vi "Autonomous Independent.vi"() -> ()   [LabVIEW 2016]
doc: "This VI is called when autonomous begins, and will automatically be terminated when autonomous ends. You can carry out timed or sensor driven robot movement independently without needing to return to the caller."
uses:
  <vilib>/Rock Robotics/Network Tables/NT Read Number.vi
  Robot Global Data.vi
  <vilib>/addons/control/pid/pid.llb/PID (DBL).vi
  <vilib>/Rock Robotics/Network Tables/NT Write Number.vi
  <vilib>/addons/control/pid/NI_PID_pid.lvlib
panel:
  out "Distance 9-2":dbl
  out "Distance 9 - 1":dbl
  out "Distance 1":dbl
  out "Distance 2":dbl
  out "Gyro Angle 4":dbl(knob) scale=0.0..360.0
  out "Gyro Zero angle":dbl
  out "Boolean 2":bool
  out "Current 2":dbl=14.75
  out "Elapsed Time (s) 2":dbl caption="Elapsed Time (s)"
  out "Boolean 9":bool
  out "Gyro Angle 4":dbl(knob) scale=0.0..360.0
  out "Numeric 2":dbl
  out "drive current 2":dbl=2.75
  out "Gyro Angle 3":dbl(knob) scale=0.0..360.0
  out "Distance 2":dbl
  out "Distance":dbl
  out "Boolean":bool
  out "Current":dbl=14.75
  out "Elapsed Time (s)":dbl
  out "Boolean 8":bool
  out "Gyro Angle 3":dbl(knob) scale=0.0..360.0
  out "Numeric":dbl
  out "drive current":dbl=2.75
  out "Gyro Angle 2":dbl(knob) scale=0.0..360.0
  out "abs(x)":dbl
  out "Loop Speed":u32
  in  "Manual Auto Select":bool
  in  "Auto Select":T1(ring)=enum."baseline"
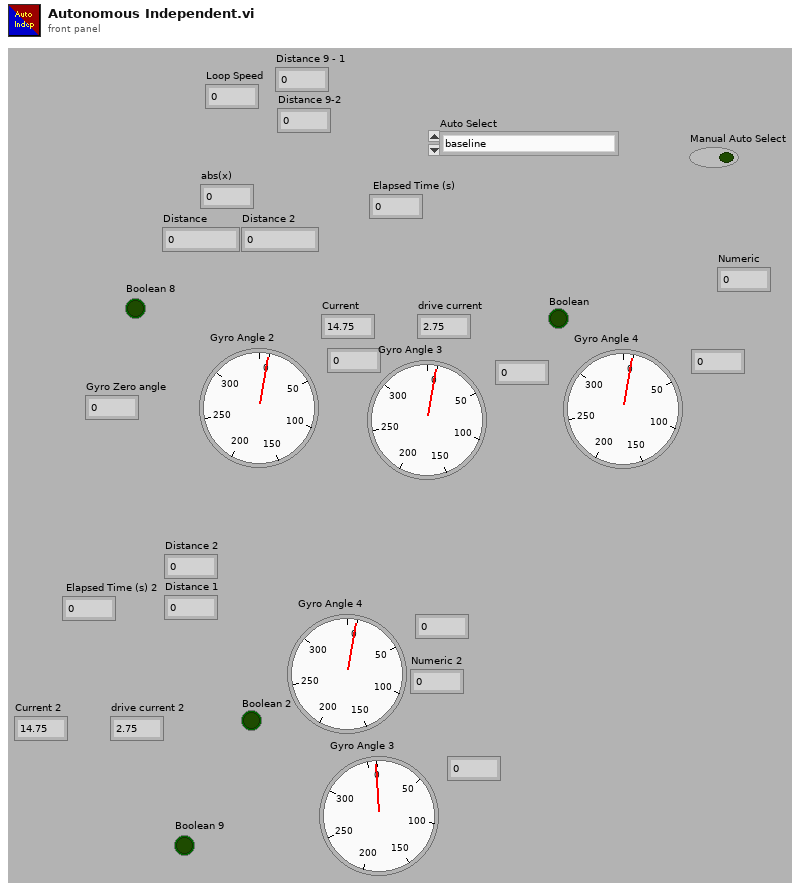
[diagram p1: front panel]
types:
  T1 = enum16{"default", "baseline", "center gear", "left gear", "right gear", "10 shoot then gear prep blue", "10 shoot then gear prep red", "Blank", "move to shoot red", "hopper shoot bue", "hopper shoot red"}
  T2 = cluster{"proportional gain (Kc)":dbl, "integral time (Ti, min)":dbl, "derivative time (Td, min)":dbl}
  T3 = typedef "WPI_EncoderDevRef.ctl" = cluster{"DevStatus":errorcluster, "EncoderIndex":T4, "CounterIndex":T5, "DistancePerCount":dbl, "Decoding Type":T6}
  T4 = typedef "FPGA_EncoderIdx.ctl" = enum8{"Enc 0", "Enc 1", "Enc 2", "Enc 3", "Enc 4", "Enc 5", "Enc 6", "Enc 7", "Invalid"}
  T5 = typedef "FPGA_CounterCtrSystemIndex.ctl" = enum8{"Ctr 0", "Ctr 1", "Ctr 2", "Ctr 3", "Ctr 4", "Ctr 5", "Ctr 6", "Ctr 7", "Invalid"}
  T6 = typedef "WPI_EncoderType.ctl" = enum16{"1x", "2x", "4x"}
  T7 = typedef "WPI_MotorControlDeviceRef.ctl" = cluster{"DeviceStatus":errorcluster, "Type":T8, "PWM":cluster{"PWM Channel":T9, "DeadBand":T10}, "CAN":cluster{"Device Number":u8, "SetOutput VI Ref":variant, "GetOutput VI Ref":variant, "Enable VI Ref":variant, "Disable VI Ref":variant, "Data":variant}, "Invert":bool}
  T8 = typedef "WPI_MotorControlType.ctl" = enum16{"PWM", "CAN"}
  T9 = typedef "FPGA_DIOPWMChannel.ctl" = enum8{"PWM 0", "PWM 1", "PWM 2", "PWM 3", "PWM 4", "PWM 5", "PWM 6", "PWM 7", "PWM 8", "PWM 9", "PWM MXP 0", "PWM MXP 1", "PWM MXP 2", "PWM MXP 3", "PWM MXP 4", "PWM MXP 5", "PWM MXP 6", "PWM MXP 7", "PWM MXP 8", "PWM MXP 9", "Invalid"}
  T10 = typedef "WPI_PWMDeadband.ctl" = cluster{"Name":string, "maxPositivePwm":i32, "minPositivePwm":i32, "centerPwm":i32, "maxNegativePwm":i32, "minNegativePwm":i32, "angularRange":u16}
  T11 = typedef "WPI_CANTalonSRX_GlobalStatus.ctl" = cluster{"Applied Throttle":dbl, "Module Enabled":bool, "CAN Error":errorcluster, "Closed Loop Error":dbl, "Forward Limit Switch Closed":bool, "Reverse Limit Switch Closed":bool, "Sensor Position":dbl, "Sensor Velocity":dbl, "Current":dbl, "Sticky Fault - Over Temp":bool, "Sticky Fault - Under Voltage":bool, "Sticky Fault - Forward Limit":bool, "Sticky Fault - Reverse Limit":bool, "Sticky Fault - Forward Soft Limit":bool, "Sticky Fault - Reverse Soft Limit":bool, "Brake is Enabled":bool, "Encoder Position":dbl, "Encoder Velocity":dbl, "Encoder Index Count":dbl, "Encoder A Pin State":bool, "Encoder B Pin State":bool, "Encoder Index Pin State":bool, "Analog In":dbl, "Analog In Velocity":dbl, "Temperature (C)":dbl, "Battery Voltage":dbl, "Control 5 Is Supported":bool, "Current Profile Slot Select":dbl, "Pos Div 8":bool, "Vel Div 4":bool, "Pulse Width Position":i32, "Pulse Width Velocity":i32, "Pulse Width Rise To Rise (us)":i32, "Pulse Width Rise To Fall (us)":i32, "Mot Prof Active Is Under Run":bool, "Mot Prof Active Has Under Run":bool, "Mot Prof Active Is Last":bool, "Mot Prof Active Velocity Only":bool, "Mot Prof Active Is Valid":bool, "Mot Prof Buffer Is Full":bool, "Mot Prof Active Profile Slot Select":i32, "Mot Prof NextID":i32, "Mot Prof Count":i32, "Mot Prof Active Velocity":dbl, "Mot Prof Active Position":dbl, "Mot Prof Output Enable":i32, "UsageFrame":u32, "Motion Magic Active Trajectory":cluster{"Velocity":dbl, "Position":dbl}}
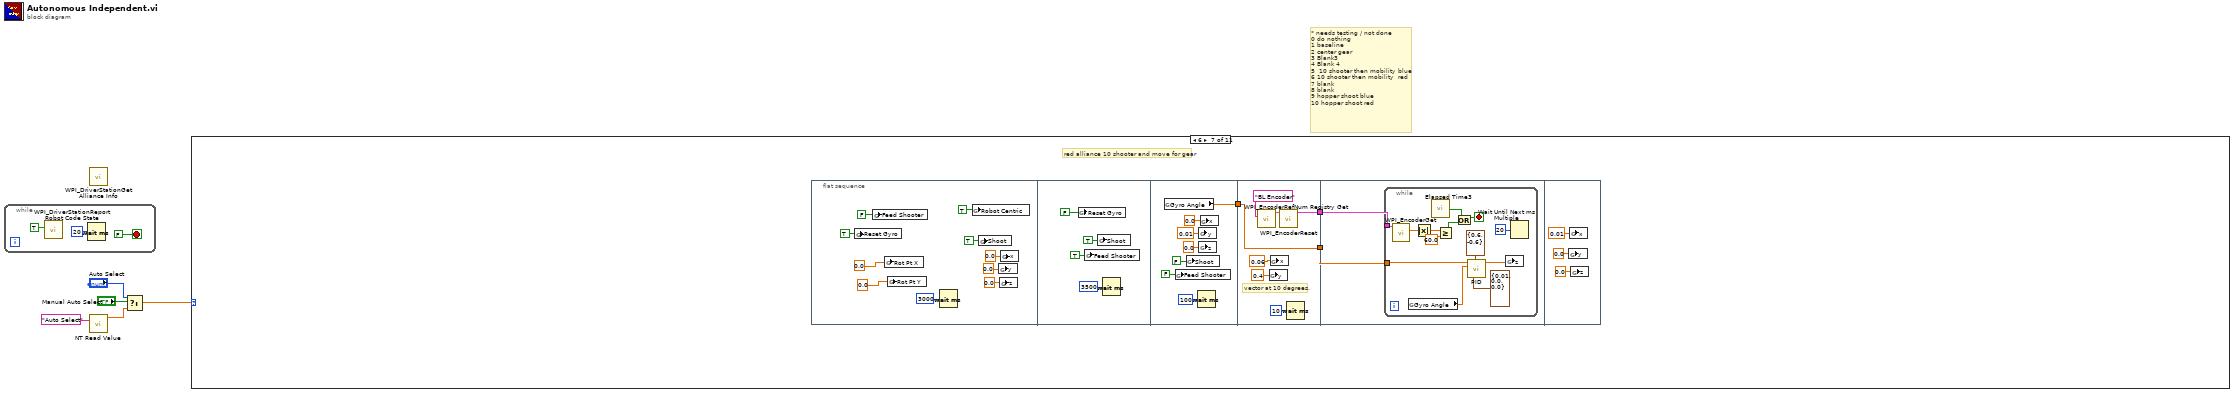
[diagram p0: block diagram]
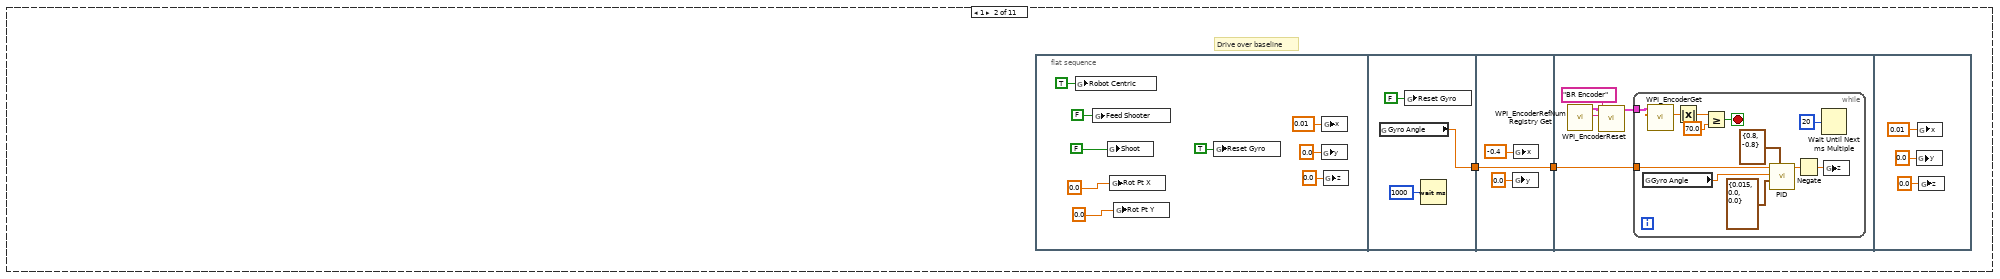
[diagram p3: hidden frame]
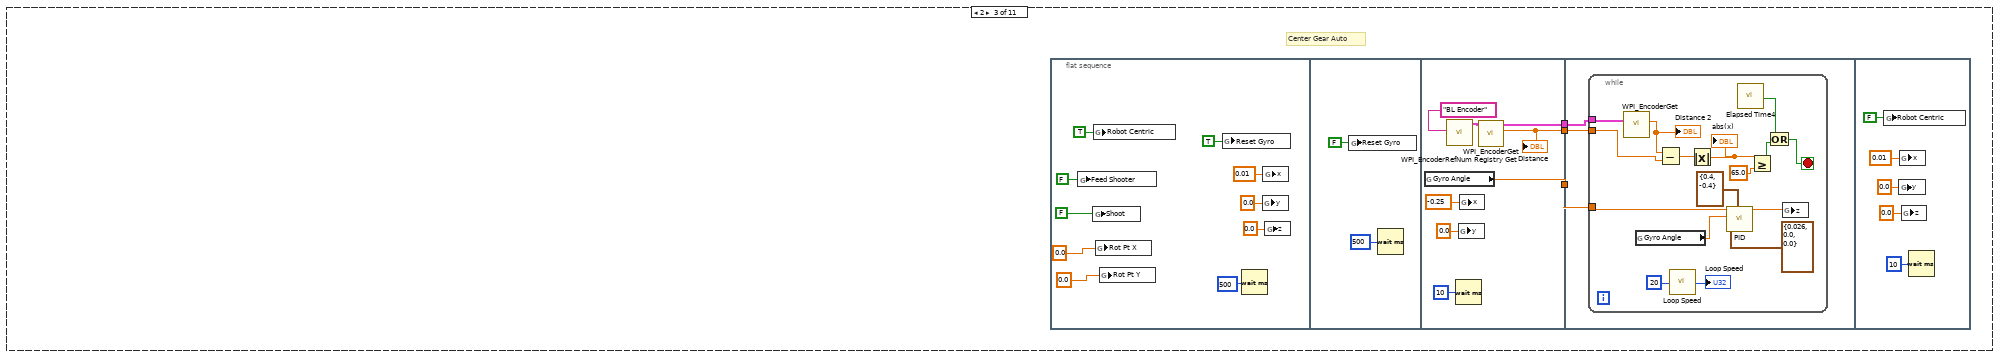
[diagram p4: hidden frame]
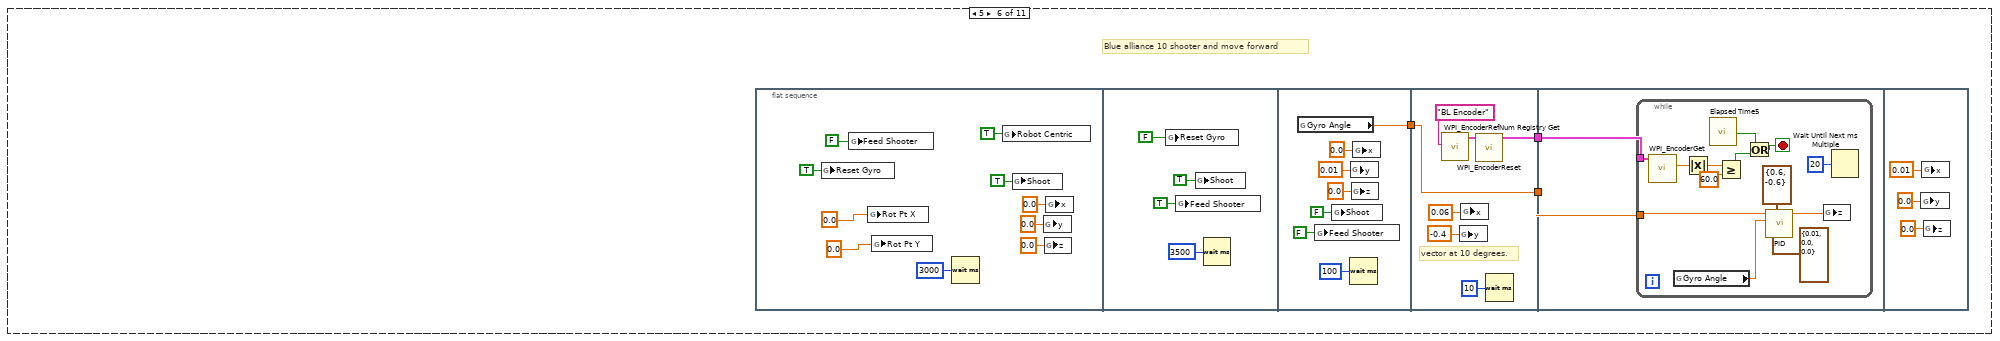
[diagram p7: hidden frame]
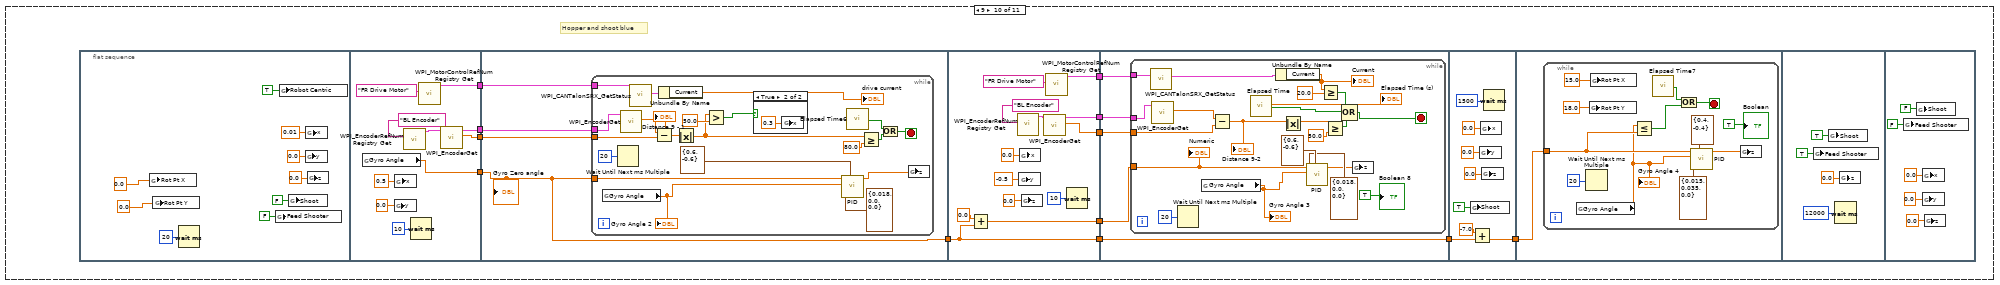
[diagram p10: hidden frame]
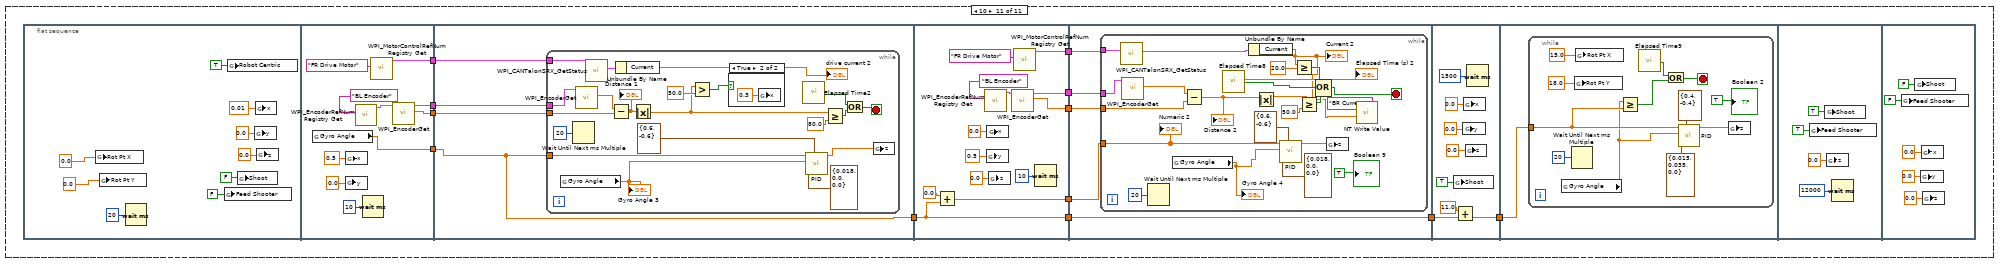
[diagram p12: hidden frame]
diagram:
  # "* needs testing / not done\n0 do nothing\n1 baseline\n2 center gear\n3 Blank3\n4 Blank 4\n5  10 shooter then mobility blue \n6 10 shooter then mobility  red\n7 blank\n8 blank\n9 hopper shoot blue\n10 hopper shoot red"
  n1 = while {
    stop <- FALSE stop-if-true
    n2 = call <vilib>:"WPI_DriverStationReport Robot Code State.vi"("Autonomous"=TRUE) -> ()  [unwired: 10 in, 1 out]
    n3 = Wait (ms)(milliseconds to wait=u32 20) -> ()  [unwired: 1 out]
  }
  n4 = call-poly <vilib>:"NT Read Value.vi"("Name"="Auto Select") -> ("Numeric"=w1:dbl)  [unwired: 9 in, 1 out]
  n5 = call <vilib>:"WPI_DriverStationGet Alliance Info.vi"() -> ()  [unwired: 12 out]
  n6 = Select(t="Auto Select", s="Manual Auto Select", f=w1) -> (s? t:f=w5:dbl)
  n7 = case shown="6" w5 {
    frame 0, Default {
    }
    frame 1 {
      # "Drive over baseline"
      n8 = flat-sequence {
        tunnel: [w21] -> w9
        tunnel: [w23] -> w10
        tunnel: w9 -> [w23]
        tunnel: w10 -> [w26]
        frame #0 {
          n9 = global write "Robot Global Data.vi" "Robot Centric"(TRUE ("Robot Centric")) -> ()
          n10 = global write "Robot Global Data.vi" "Feed Shooter"(FALSE ("Robot Centric")) -> ()
          n11 = global write "Robot Global Data.vi" "Shoot"(FALSE ("Robot Centric")) -> ()
          n12 = global write "Robot Global Data.vi" "Rot Pt X"(0.0 ("Rot Pt X")) -> ()
          n13 = global write "Robot Global Data.vi" "Rot Pt Y"(0.0 ("Rot Pt X")) -> ()
          n14 = global write "Robot Global Data.vi" "Reset Gyro"(TRUE ("Reset Gyro")) -> ()
          n15 = global write "Robot Global Data.vi" "y"(0.0 ("y")) -> ()
          n16 = global write "Robot Global Data.vi" "x"(0.01 ("x")) -> ()
          n17 = global write "Robot Global Data.vi" "z"(0.0 ("z")) -> ()
        }
        frame #1 {
          n18 = global read "Robot Global Data.vi" "Gyro Angle"() -> (w21:dbl)
          n19 = global write "Robot Global Data.vi" "Reset Gyro"(FALSE ("Reset Gyro")) -> ()
          n20 = Wait (ms)(milliseconds to wait=u32 1000) -> ()  [unwired: 1 out]
        }
        frame #2 {
          n21 = global write "Robot Global Data.vi" "y"(0.0 ("y")) -> ()
          n22 = global write "Robot Global Data.vi" "x"(-0.4 ("x")) -> ()
        }
        frame #3 {
          n23 = call <vilib>:"WPI_EncoderRefNum Registry Get.vi"("refnum name"="BR Encoder") -> ("EncoderDevRef"=w28:T3)  [unwired: 9 in, 1 out]
          n24 = call <vilib>:"WPI_EncoderReset.vi"("EncoderDevRef"=w28) -> ("EncoderDevRef"=w27:T3)  [unwired: 9 in, 1 out]
          n25 = while {
            tunnel: w27 -> [w41]
            tunnel: w26 -> [w32]
            stop <- w39 stop-if-true
            n26 = global read "Robot Global Data.vi" "Gyro Angle"() -> (w31:dbl)
            n27 = call <vilib>:"WPI_EncoderGet.vi"("EncoderDevRef"=w41) -> ("Distance"=w40:dbl)  [unwired: 5 in, 5 out]
            n28 = Absolute Value(x=w40) -> (abs(x)=w34:dbl)
            n29 = Greater Or Equal?(x=w34, y=70.0) -> (x >= y?=w39:bool)
            n30 = call-poly <vilib>:"PID.vi"("output range"=cluster{"output high":dbl, "output low":dbl} {"output high"=0.8, "output low"=-0.8}, "PID gains"=T2 {"proportional gain (Kc)"=0.015, "integral time (Ti, min)"=0.0, "derivative time (Td, min)"=0.0} ("PID gains 2"), "process variable"=w31, "setpoint"=w32) -> ("output"=w37:dbl)  [unwired: 6 in, 1 out]
            n31 = Negate(x=w37) -> (-x=w35:dbl)
            n32 = Wait Until Next ms Multiple(millisecond multiple=u32 20) -> ()  [unwired: 1 out]
            n33 = global write "Robot Global Data.vi" "z"(w35) -> ()
          }
        }
        frame #4 {
          n34 = global write "Robot Global Data.vi" "y"(0.0 ("y")) -> ()
          n35 = global write "Robot Global Data.vi" "x"(0.01 ("x")) -> ()
          n36 = global write "Robot Global Data.vi" "z"(0.0 ("z")) -> ()
        }
      }
    }
    frame 2 {
      # "Center Gear Auto"
      n37 = flat-sequence {
        tunnel: [w65] -> w47
        tunnel: [w61] -> w46
        tunnel: [w60] -> w45
        tunnel: w47 -> [w70]
        tunnel: w46 -> [w69]
        tunnel: w45 -> [w68]
        frame #0 {
          n38 = global write "Robot Global Data.vi" "Feed Shooter"(FALSE ("Robot Centric")) -> ()
          n39 = global write "Robot Global Data.vi" "Shoot"(FALSE ("Robot Centric")) -> ()
          n40 = global write "Robot Global Data.vi" "Robot Centric"(TRUE ("Robot Centric")) -> ()
          n41 = global write "Robot Global Data.vi" "Rot Pt X"(0.0 ("Rot Pt X")) -> ()
          n42 = global write "Robot Global Data.vi" "Rot Pt Y"(0.0 ("Rot Pt X")) -> ()
          n43 = global write "Robot Global Data.vi" "Reset Gyro"(TRUE ("Reset Gyro")) -> ()
          n44 = Wait (ms)(milliseconds to wait=u32 500) -> ()  [unwired: 1 out]
          n45 = global write "Robot Global Data.vi" "y"(0.0 ("y")) -> ()
          n46 = global write "Robot Global Data.vi" "x"(0.01 ("x")) -> ()
          n47 = global write "Robot Global Data.vi" "z"(0.0 ("z")) -> ()
        }
        frame #1 {
          n48 = global write "Robot Global Data.vi" "Reset Gyro"(FALSE ("Reset Gyro")) -> ()
          n49 = Wait (ms)(milliseconds to wait=u32 500) -> ()  [unwired: 1 out]
        }
        frame #2 {
          n50 = global read "Robot Global Data.vi" "Gyro Angle"() -> (w65:dbl)
          n51 = call <vilib>:"WPI_EncoderRefNum Registry Get.vi"("refnum name"="BL Encoder") -> ("EncoderDevRef"=w63:T3)  [unwired: 9 in, 1 out]
          n52 = Wait (ms)(milliseconds to wait=u32 10) -> ()  [unwired: 1 out]
          n53 = global write "Robot Global Data.vi" "y"(0.0 ("y")) -> ()
          n54 = global write "Robot Global Data.vi" "x"(-0.25 ("x")) -> ()
          n55 = call <vilib>:"WPI_EncoderGet.vi"("EncoderDevRef"=w63) -> ("Distance"=w60:dbl, "EncoderDevRef"=w61:T3)  [unwired: 5 in, 4 out]
          "Distance" <- w60
        }
        frame #3 {
          n56 = while {
            tunnel: w69 -> [w86]
            tunnel: w70 -> [w83]
            tunnel: w68 -> [w76]
            stop <- w71 stop-if-true
            n57 = call <vilib>:"WPI_EncoderGet.vi"("EncoderDevRef"=w86) -> ("Distance"=w77:dbl)  [unwired: 5 in, 5 out]
            "Distance 2" <- w77
            n58 = global read "Robot Global Data.vi" "Gyro Angle"() -> (w81:dbl)
            n59 = Subtract(x=w77, y=w76) -> (x-y=w75:dbl)
            n60 = call "Loop Speed.vi"("milliseconds to wait"=u32 20) -> ("Loop Speed"=→"Loop Speed":u32)
            n61 = Absolute Value(x=w75) -> (abs(x)=w74:dbl)
            "abs(x)" <- w74
            n62 = call-poly <vilib>:"PID.vi"("output range"=cluster{"output high":dbl, "output low":dbl} {"output high"=0.4, "output low"=-0.4}, "PID gains"=T2 {"proportional gain (Kc)"=0.026, "integral time (Ti, min)"=0.0, "derivative time (Td, min)"=0.0}, "process variable"=w81, "setpoint"=w83) -> ("output"=w79:dbl)  [unwired: 6 in, 1 out]
            n63 = call "Elapsed Time4"() -> ("Time has Elapsed"=w72:bool)  [unwired: 12 in, 7 out]
            n64 = Greater Or Equal?(x=w74, y=65.0) -> (x >= y?=w73:bool)
            n65 = Or(x=w72, y=w73) -> (x .or. y?=w71:bool)
            n66 = global write "Robot Global Data.vi" "z"(w79) -> ()
          }
        }
        frame #4 {
          n67 = global write "Robot Global Data.vi" "Robot Centric"(FALSE ("Robot Centric")) -> ()
          n68 = global write "Robot Global Data.vi" "y"(0.0 ("y")) -> ()
          n69 = global write "Robot Global Data.vi" "x"(0.01 ("x")) -> ()
          n70 = global write "Robot Global Data.vi" "z"(0.0 ("z")) -> ()
          n71 = Wait (ms)(milliseconds to wait=u32 10) -> ()  [unwired: 1 out]
        }
      }
    }
    frame 3 {
      # "find current of drive motors when\n they have more than normal load\n and use that as a safe stop"
    }
    frame 4 {
    }
    frame 5 {
      # "Blue alliance 10 shooter and move forward"
      n72 = flat-sequence {
        tunnel: [w109] -> w93
        tunnel: [w120] -> w94
        tunnel: w93 -> [w120]
        tunnel: [w117] -> w92
        tunnel: w94 -> [w124]
        tunnel: w92 -> [w123]
        frame #0 {
          n73 = global write "Robot Global Data.vi" "Reset Gyro"(TRUE ("Reset Gyro")) -> ()
          n74 = global write "Robot Global Data.vi" "Feed Shooter"(FALSE ("Robot Centric")) -> ()
          n75 = global write "Robot Global Data.vi" "Rot Pt X"(0.0 ("Rot Pt X")) -> ()
          n76 = global write "Robot Global Data.vi" "Rot Pt Y"(0.0 ("Rot Pt X")) -> ()
          n77 = Wait (ms)(milliseconds to wait=u32 3000) -> ()  [unwired: 1 out]
          n78 = global write "Robot Global Data.vi" "Robot Centric"(TRUE ("Robot Centric")) -> ()
          n79 = global write "Robot Global Data.vi" "Shoot"(TRUE ("Shoot")) -> ()
          n80 = global write "Robot Global Data.vi" "y"(0.0 ("y")) -> ()
          n81 = global write "Robot Global Data.vi" "z"(0.0 ("z")) -> ()
          n82 = global write "Robot Global Data.vi" "x"(0.0 ("x")) -> ()
        }
        frame #1 {
          n83 = global write "Robot Global Data.vi" "Reset Gyro"(FALSE ("Reset Gyro")) -> ()
          n84 = global write "Robot Global Data.vi" "Feed Shooter"(TRUE ("Feed Shooter")) -> ()
          n85 = global write "Robot Global Data.vi" "Shoot"(TRUE ("Shoot")) -> ()
          n86 = Wait (ms)(milliseconds to wait=u32 3500) -> ()  [unwired: 1 out]
        }
        frame #2 {
          n87 = global read "Robot Global Data.vi" "Gyro Angle"() -> (w109:dbl)
          n88 = global write "Robot Global Data.vi" "Feed Shooter"(FALSE ("Feed Shooter")) -> ()
          n89 = global write "Robot Global Data.vi" "Shoot"(FALSE ("Shoot")) -> ()
          n90 = Wait (ms)(milliseconds to wait=u32 100) -> ()  [unwired: 1 out]
          n91 = global write "Robot Global Data.vi" "y"(0.01 ("y")) -> ()
          n92 = global write "Robot Global Data.vi" "z"(0.0 ("z")) -> ()
          n93 = global write "Robot Global Data.vi" "x"(0.0 ("x")) -> ()
        }
        frame #3 {
          # "vector at 10 degrees."
          n94 = call <vilib>:"WPI_EncoderRefNum Registry Get.vi"("refnum name"="BL Encoder") -> ("EncoderDevRef"=w118:T3)  [unwired: 9 in, 1 out]
          n95 = global write "Robot Global Data.vi" "y"(-0.4 ("y")) -> ()
          n96 = global write "Robot Global Data.vi" "x"(0.06 ("x")) -> ()
          n97 = call <vilib>:"WPI_EncoderReset.vi"("EncoderDevRef"=w118) -> ("EncoderDevRef"=w117:T3)  [unwired: 9 in, 1 out]
          n98 = Wait (ms)(milliseconds to wait=u32 10) -> ()  [unwired: 1 out]
        }
        frame #4 {
          n99 = while {
            tunnel: w123 -> [w137]
            tunnel: w124 -> [w133]
            stop <- w128 stop-if-true
            n100 = call <vilib>:"WPI_EncoderGet.vi"("EncoderDevRef"=w137) -> ("Distance"=w136:dbl)  [unwired: 5 in, 5 out]
            n101 = global read "Robot Global Data.vi" "Gyro Angle"() -> (w130:dbl)
            n102 = Absolute Value(x=w136) -> (abs(x)=w132:dbl)
            n103 = call "Elapsed Time5"() -> ("Time has Elapsed"=w126:bool)  [unwired: 12 in, 7 out]
            n104 = Greater Or Equal?(x=w132, y=60.0 ("Distance to travel")) -> (x >= y?=w127:bool)
            n105 = Or(x=w126, y=w127) -> (x .or. y?=w128:bool)
            n106 = call-poly <vilib>:"PID.vi"("output range"=cluster{"output high":dbl, "output low":dbl} {"output high"=0.6, "output low"=-0.6}, "PID gains"=T2 {"proportional gain (Kc)"=0.01, "integral time (Ti, min)"=0.0, "derivative time (Td, min)"=0.0}, "process variable"=w130, "setpoint"=w133) -> ("output"=w125:dbl)  [unwired: 6 in, 1 out]
            n107 = global write "Robot Global Data.vi" "z"(w125) -> ()
            n108 = Wait Until Next ms Multiple(millisecond multiple=u32 20) -> ()  [unwired: 1 out]
          }
        }
        frame #5 {
          n109 = global write "Robot Global Data.vi" "y"(0.0 ("y")) -> ()
          n110 = global write "Robot Global Data.vi" "x"(0.01 ("x")) -> ()
          n111 = global write "Robot Global Data.vi" "z"(0.0 ("z")) -> ()
        }
      }
    }
    frame 6 {
      # "red alliance 10 shooter and move for gear"
      n112 = flat-sequence {
        tunnel: [w158] -> w143
        tunnel: [w169] -> w142
        tunnel: w143 -> [w169]
        tunnel: [w166] -> w141
        tunnel: w142 -> [w172]
        tunnel: w141 -> [w173]
        frame #0 {
          n113 = global write "Robot Global Data.vi" "Reset Gyro"(TRUE ("Reset Gyro")) -> ()
          n114 = global write "Robot Global Data.vi" "Feed Shooter"(FALSE ("Robot Centric")) -> ()
          n115 = global write "Robot Global Data.vi" "Rot Pt X"(0.0 ("Rot Pt X")) -> ()
          n116 = global write "Robot Global Data.vi" "Rot Pt Y"(0.0 ("Rot Pt X")) -> ()
          n117 = Wait (ms)(milliseconds to wait=u32 3000) -> ()  [unwired: 1 out]
          n118 = global write "Robot Global Data.vi" "Robot Centric"(TRUE ("Robot Centric")) -> ()
          n119 = global write "Robot Global Data.vi" "Shoot"(TRUE ("Shoot")) -> ()
          n120 = global write "Robot Global Data.vi" "y"(0.0 ("y")) -> ()
          n121 = global write "Robot Global Data.vi" "z"(0.0 ("z")) -> ()
          n122 = global write "Robot Global Data.vi" "x"(0.0 ("x")) -> ()
        }
        frame #1 {
          n123 = global write "Robot Global Data.vi" "Reset Gyro"(FALSE ("Reset Gyro")) -> ()
          n124 = global write "Robot Global Data.vi" "Feed Shooter"(TRUE ("Feed Shooter")) -> ()
          n125 = global write "Robot Global Data.vi" "Shoot"(TRUE ("Shoot")) -> ()
          n126 = Wait (ms)(milliseconds to wait=u32 3500) -> ()  [unwired: 1 out]
        }
        frame #2 {
          n127 = global read "Robot Global Data.vi" "Gyro Angle"() -> (w158:dbl)
          n128 = global write "Robot Global Data.vi" "Feed Shooter"(FALSE ("Feed Shooter")) -> ()
          n129 = global write "Robot Global Data.vi" "Shoot"(FALSE ("Shoot")) -> ()
          n130 = Wait (ms)(milliseconds to wait=u32 100) -> ()  [unwired: 1 out]
          n131 = global write "Robot Global Data.vi" "y"(0.01 ("y")) -> ()
          n132 = global write "Robot Global Data.vi" "z"(0.0 ("z")) -> ()
          n133 = global write "Robot Global Data.vi" "x"(0.0 ("x")) -> ()
        }
        frame #3 {
          # "vector at 10 degrees."
          n134 = call <vilib>:"WPI_EncoderRefNum Registry Get.vi"("refnum name"="BL Encoder") -> ("EncoderDevRef"=w167:T3)  [unwired: 9 in, 1 out]
          n135 = global write "Robot Global Data.vi" "y"(0.4 ("y")) -> ()
          n136 = global write "Robot Global Data.vi" "x"(0.06 ("x")) -> ()
          n137 = call <vilib>:"WPI_EncoderReset.vi"("EncoderDevRef"=w167) -> ("EncoderDevRef"=w166:T3)  [unwired: 9 in, 1 out]
          n138 = Wait (ms)(milliseconds to wait=u32 10) -> ()  [unwired: 1 out]
        }
        frame #4 {
          n139 = while {
            tunnel: w173 -> [w186]
            tunnel: w172 -> [w182]
            stop <- w177 stop-if-true
            n140 = call <vilib>:"WPI_EncoderGet.vi"("EncoderDevRef"=w186) -> ("Distance"=w185:dbl)  [unwired: 5 in, 5 out]
            n141 = global read "Robot Global Data.vi" "Gyro Angle"() -> (w179:dbl)
            n142 = Absolute Value(x=w185) -> (abs(x)=w181:dbl)
            n143 = call "Elapsed Time3"() -> ("Time has Elapsed"=w175:bool)  [unwired: 12 in, 7 out]
            n144 = Greater Or Equal?(x=w181, y=60.0 ("Distance to travel")) -> (x >= y?=w176:bool)
            n145 = Or(x=w175, y=w176) -> (x .or. y?=w177:bool)
            n146 = call-poly <vilib>:"PID.vi"("output range"=cluster{"output high":dbl, "output low":dbl} {"output high"=0.6, "output low"=-0.6}, "PID gains"=T2 {"proportional gain (Kc)"=0.01, "integral time (Ti, min)"=0.0, "derivative time (Td, min)"=0.0}, "process variable"=w179, "setpoint"=w182) -> ("output"=w174:dbl)  [unwired: 6 in, 1 out]
            n147 = global write "Robot Global Data.vi" "z"(w174) -> ()
            n148 = Wait Until Next ms Multiple(millisecond multiple=u32 20) -> ()  [unwired: 1 out]
          }
        }
        frame #5 {
          n149 = global write "Robot Global Data.vi" "y"(0.0 ("y")) -> ()
          n150 = global write "Robot Global Data.vi" "x"(0.01 ("x")) -> ()
          n151 = global write "Robot Global Data.vi" "z"(0.0 ("z")) -> ()
        }
      }
    }
    frame 7 {
    }
    frame 8 {
    }
    frame 9 {
      # "Hopper and shoot blue"
      n152 = flat-sequence {
        tunnel: [w219] -> w194
        tunnel: [w213] -> w193
        tunnel: [w212] -> w192
        tunnel: [w211] -> w191
        tunnel: w194 -> [w224]
        tunnel: [w224] -> w201
        tunnel: w193 -> [w223]
        tunnel: w192 -> [w222]
        tunnel: w191 -> [w221]
        tunnel: w201 -> [w256]
        tunnel: [w257] -> w200
        tunnel: [w256] -> w199
        tunnel: [w249] -> w196
        tunnel: [w248] -> w195
        tunnel: [w246] -> w190
        tunnel: w200 -> [w263]
        tunnel: [w262] -> w198
        tunnel: w199 -> [w262]
        tunnel: w196 -> [w261]
        tunnel: w195 -> [w260]
        tunnel: w190 -> [w259]
        tunnel: [w289] -> w197
        tunnel: w198 -> [w290]
        tunnel: w197 -> [w294]
        frame #0 {
          n153 = global write "Robot Global Data.vi" "Rot Pt X"(0.0 ("Rot Pt X")) -> ()
          n154 = global write "Robot Global Data.vi" "Rot Pt Y"(0.0 ("Rot Pt X")) -> ()
          n155 = Wait (ms)(milliseconds to wait=u32 20) -> ()  [unwired: 1 out]
          n156 = global write "Robot Global Data.vi" "Feed Shooter"(FALSE ("Feed Shooter")) -> ()
          n157 = global write "Robot Global Data.vi" "Robot Centric"(TRUE ("Robot Centric")) -> ()
          n158 = global write "Robot Global Data.vi" "Shoot"(FALSE ("Shoot")) -> ()
          n159 = global write "Robot Global Data.vi" "y"(0.0 ("y")) -> ()
          n160 = global write "Robot Global Data.vi" "x"(0.01 ("x")) -> ()
          n161 = global write "Robot Global Data.vi" "z"(0.0 ("z")) -> ()
        }
        frame #1 {
          n162 = global read "Robot Global Data.vi" "Gyro Angle"() -> (w219:dbl)
          n163 = global write "Robot Global Data.vi" "y"(0.0 ("y")) -> ()
          n164 = global write "Robot Global Data.vi" "x"(0.5 ("x")) -> ()
          n165 = call <vilib>:"WPI_EncoderRefNum Registry Get.vi"("refnum name"="BL Encoder") -> ("EncoderDevRef"=w215:T3)  [unwired: 9 in, 1 out]
          n166 = Wait (ms)(milliseconds to wait=u32 10) -> ()  [unwired: 1 out]
          n167 = call <vilib>:"WPI_MotorControlRefNum Registry Get.vi"("refnum name"="FR Drive Motor") -> ("MotorControlDevRef"=w211:T7)  [unwired: 9 in, 1 out]
          n168 = call <vilib>:"WPI_EncoderGet.vi"("EncoderDevRef"=w215) -> ("Distance"=w213:dbl, "EncoderDevRef"=w212:T3)  [unwired: 5 in, 4 out]
        }
        frame #2 {
          n169 = while {
            tunnel: w224 -> [w242]
            tunnel: w223 -> [w231]
            tunnel: w222 -> [w230]
            tunnel: w221 -> [w229]
            stop <- w233 stop-if-true
            n170 = global read "Robot Global Data.vi" "Gyro Angle"() -> (w238:dbl)
            "Gyro Angle 2" <- w238
            n171 = Wait Until Next ms Multiple(millisecond multiple=u32 20) -> ()  [unwired: 1 out]
            n172 = call <vilib>:"WPI_EncoderGet.vi"("EncoderDevRef"=w230) -> ("Distance"=w232:dbl)  [unwired: 5 in, 5 out]
            n173 = call <vilib>:"WPI_CANTalonSRX_GetStatus.vi"("CAN Talon SRX Ref"=w229) -> ("Talon SRX Status"=w240:T11)  [unwired: 8 in, 2 out]
            n174 = Subtract(x=w232, y=w231) -> (x-y=w228:dbl)
            "Distance 9 - 1" <- w228
            n175 = Unbundle By Name(w240) -> ("Current"=→"drive current":dbl)
            n176 = Absolute Value(x=w228) -> (abs(x)=w225:dbl)
            n177 = Greater?(x=w225, y=50.0) -> (0:w226:bool)
            n178 = case shown="True" w226 {
              frame False {
              }
              frame True {
                n179 = global write "Robot Global Data.vi" "x"(0.3 ("x")) -> ()
              }
            }
            n180 = call-poly <vilib>:"PID.vi"("output range"=cluster{"output high":dbl, "output low":dbl} {"output high"=0.6, "output low"=-0.6}, "PID gains"=T2 {"proportional gain (Kc)"=0.018, "integral time (Ti, min)"=0.0, "derivative time (Td, min)"=0.0}, "process variable"=w238, "setpoint"=w242) -> ("output"=w236:dbl)  [unwired: 6 in, 1 out]
            n181 = call "Elapsed Time6"() -> ("Time has Elapsed"=w234:bool)  [unwired: 12 in, 7 out]
            n182 = Greater Or Equal?(x=w225, y=80.0) -> (x >= y?=w235:bool)
            n183 = Or(x=w234, y=w235) -> (x .or. y?=w233:bool)
            n184 = global write "Robot Global Data.vi" "z"(w236) -> ()
          }
          "Gyro Zero angle" <- w224
        }
        frame #3 {
          n185 = Add(x=0.0, y=w256) -> (x+y=w257:dbl)
          n186 = call <vilib>:"WPI_EncoderRefNum Registry Get.vi"("refnum name"="BL Encoder") -> ("EncoderDevRef"=w251:T3)  [unwired: 9 in, 1 out]
          n187 = global write "Robot Global Data.vi" "y"(-0.5 ("y")) -> ()
          n188 = global write "Robot Global Data.vi" "x"(0.0 ("x")) -> ()
          n189 = global write "Robot Global Data.vi" "z"(0.0 ("z")) -> ()
          n190 = call <vilib>:"WPI_EncoderGet.vi"("EncoderDevRef"=w251) -> ("Distance"=w246:dbl, "EncoderDevRef"=w249:T3)  [unwired: 5 in, 4 out]
          n191 = call <vilib>:"WPI_MotorControlRefNum Registry Get.vi"("refnum name"="FR Drive Motor") -> ("MotorControlDevRef"=w248:T7)  [unwired: 9 in, 1 out]
          n192 = Wait (ms)(milliseconds to wait=u32 10) -> ()  [unwired: 1 out]
        }
        frame #4 {
          n193 = while {
            tunnel: w261 -> [w285]
            tunnel: w263 -> [w282]
            tunnel: w260 -> [w278]
            tunnel: w259 -> [w264]
            stop <- w274 stop-if-true
            n194 = call <vilib>:"WPI_CANTalonSRX_GetStatus.vi"("CAN Talon SRX Ref"=w278) -> ("Talon SRX Status"=w279:T11)  [unwired: 8 in, 2 out]
            n195 = call <vilib>:"WPI_EncoderGet.vi"("EncoderDevRef"=w285) -> ("Distance"=w265:dbl)  [unwired: 5 in, 5 out]
            n196 = Wait Until Next ms Multiple(millisecond multiple=u32 20) -> ()  [unwired: 1 out]
            n197 = global read "Robot Global Data.vi" "Gyro Angle"() -> (w267:dbl)
            "Gyro Angle 3" <- w267
            n198 = Subtract(x=w265, y=w264) -> (x-y=w266:dbl)
            "Distance 9-2" <- w266
            n199 = call "Elapsed Time"() -> ("Elapsed Time (s)"=→"Elapsed Time (s)":dbl, "Time has Elapsed"=w272:bool)  [unwired: 12 in, 6 out]
            n200 = Unbundle By Name(w279) -> ("Current"=w273:dbl)
            "Current" <- w273
            n201 = Absolute Value(x=w266) -> (abs(x)=w281:dbl)
            n202 = call-poly <vilib>:"PID.vi"("output range"=cluster{"output high":dbl, "output low":dbl} {"output high"=0.6, "output low"=-0.6}, "PID gains"=T2 {"proportional gain (Kc)"=0.018, "integral time (Ti, min)"=0.0, "derivative time (Td, min)"=0.0}, "process variable"=w267, "setpoint"=w282) -> ("output"=w268:dbl)  [unwired: 6 in, 1 out]
            n203 = Greater Or Equal?(x=w273, y=20.0) -> (x >= y?=w275:bool)
            n204 = Greater Or Equal?(x=w281, y=50.0) -> (x >= y?=w276:bool)
            n205 = Compound Arithmetic op=OR(w272, w275, w276) -> (w274:bool)
            n206 = global write "Robot Global Data.vi" "z"(w268) -> ()
            "Boolean 8" <- TRUE
            "Numeric" <- w282
          }
        }
        frame #5 {
          n207 = global write "Robot Global Data.vi" "Shoot"(TRUE ("Shoot")) -> ()
          n208 = Add(x=-7.0, y=w290) -> (x+y=w289:dbl)
          n209 = global write "Robot Global Data.vi" "y"(0.0 ("y")) -> ()
          n210 = global write "Robot Global Data.vi" "x"(0.0 ("x")) -> ()
          n211 = global write "Robot Global Data.vi" "z"(0.0 ("z")) -> ()
          n212 = Wait (ms)(milliseconds to wait=u32 1500) -> ()  [unwired: 1 out]
        }
        frame #6 {
          n213 = while {
            tunnel: w294 -> [w304]
            stop <- w297 stop-if-true
            n214 = global read "Robot Global Data.vi" "Gyro Angle"() -> (w295:dbl)
            "Gyro Angle 4" <- w295
            n215 = Wait Until Next ms Multiple(millisecond multiple=u32 20) -> ()  [unwired: 1 out]
            n216 = global write "Robot Global Data.vi" "Rot Pt Y"(18.0 ("x")) -> ()
            n217 = global write "Robot Global Data.vi" "Rot Pt X"(15.0 ("x")) -> ()
            n218 = Less Or Equal?(x=w295, y=w304) -> (x <= y?=w298:bool)
            n219 = call "Elapsed Time7"() -> ("Time has Elapsed"=w296:bool)  [unwired: 12 in, 7 out]
            n220 = Or(x=w296, y=w298) -> (x .or. y?=w297:bool)
            n221 = call-poly <vilib>:"PID.vi"("output range"=cluster{"output high":dbl, "output low":dbl} {"output high"=0.4, "output low"=-0.4}, "PID gains"=T2 {"proportional gain (Kc)"=0.015, "integral time (Ti, min)"=0.035, "derivative time (Td, min)"=0.0} ("PID gains 2"), "process variable"=w295, "setpoint"=w304) -> ("output"=w299:dbl)  [unwired: 6 in, 1 out]
            n222 = global write "Robot Global Data.vi" "z"(w299) -> ()
            "Boolean" <- TRUE
          }
        }
        frame #7 {
          n223 = global write "Robot Global Data.vi" "Feed Shooter"(TRUE ("Feed Shooter")) -> ()
          n224 = global write "Robot Global Data.vi" "Shoot"(TRUE ("Shoot")) -> ()
          n225 = Wait (ms)(milliseconds to wait=u32 12000) -> ()  [unwired: 1 out]
          n226 = global write "Robot Global Data.vi" "z"(0.0 ("z")) -> ()
        }
        frame #8 {
          n227 = global write "Robot Global Data.vi" "Feed Shooter"(FALSE ("Feed Shooter")) -> ()
          n228 = global write "Robot Global Data.vi" "Shoot"(FALSE ("Shoot")) -> ()
          n229 = global write "Robot Global Data.vi" "y"(0.0 ("y")) -> ()
          n230 = global write "Robot Global Data.vi" "x"(0.0 ("x")) -> ()
          n231 = global write "Robot Global Data.vi" "z"(0.0 ("z")) -> ()
        }
      }
    }
    frame 10 {
      n232 = flat-sequence {
        tunnel: [w345] -> w327
        tunnel: [w339] -> w326
        tunnel: [w338] -> w325
        tunnel: [w337] -> w324
        tunnel: w327 -> [w350]
        tunnel: [w350] -> w323
        tunnel: w326 -> [w349]
        tunnel: w325 -> [w348]
        tunnel: w324 -> [w347]
        tunnel: w323 -> [w382]
        tunnel: [w383] -> w322
        tunnel: [w382] -> w321
        tunnel: [w375] -> w320
        tunnel: [w374] -> w319
        tunnel: [w372] -> w318
        tunnel: w322 -> [w389]
        tunnel: [w388] -> w317
        tunnel: w321 -> [w388]
        tunnel: w320 -> [w387]
        tunnel: w319 -> [w386]
        tunnel: w318 -> [w385]
        tunnel: [w416] -> w316
        tunnel: w317 -> [w417]
        tunnel: w316 -> [w421]
        frame #0 {
          n233 = global write "Robot Global Data.vi" "Rot Pt X"(0.0 ("Rot Pt X")) -> ()
          n234 = global write "Robot Global Data.vi" "Rot Pt Y"(0.0 ("Rot Pt X")) -> ()
          n235 = Wait (ms)(milliseconds to wait=u32 20) -> ()  [unwired: 1 out]
          n236 = global write "Robot Global Data.vi" "Feed Shooter"(FALSE ("Feed Shooter")) -> ()
          n237 = global write "Robot Global Data.vi" "Robot Centric"(TRUE ("Robot Centric")) -> ()
          n238 = global write "Robot Global Data.vi" "Shoot"(FALSE ("Shoot")) -> ()
          n239 = global write "Robot Global Data.vi" "y"(0.0 ("y")) -> ()
          n240 = global write "Robot Global Data.vi" "x"(0.01 ("x")) -> ()
          n241 = global write "Robot Global Data.vi" "z"(0.0 ("z")) -> ()
        }
        frame #1 {
          n242 = global read "Robot Global Data.vi" "Gyro Angle"() -> (w345:dbl)
          n243 = global write "Robot Global Data.vi" "y"(0.0 ("y")) -> ()
          n244 = global write "Robot Global Data.vi" "x"(0.5 ("x")) -> ()
          n245 = call <vilib>:"WPI_EncoderRefNum Registry Get.vi"("refnum name"="BL Encoder") -> ("EncoderDevRef"=w341:T3)  [unwired: 9 in, 1 out]
          n246 = Wait (ms)(milliseconds to wait=u32 10) -> ()  [unwired: 1 out]
          n247 = call <vilib>:"WPI_MotorControlRefNum Registry Get.vi"("refnum name"="FR Drive Motor") -> ("MotorControlDevRef"=w337:T7)  [unwired: 9 in, 1 out]
          n248 = call <vilib>:"WPI_EncoderGet.vi"("EncoderDevRef"=w341) -> ("Distance"=w339:dbl, "EncoderDevRef"=w338:T3)  [unwired: 5 in, 4 out]
        }
        frame #2 {
          n249 = while {
            tunnel: w350 -> [w368]
            tunnel: w349 -> [w357]
            tunnel: w348 -> [w356]
            tunnel: w347 -> [w355]
            stop <- w359 stop-if-true
            n250 = global read "Robot Global Data.vi" "Gyro Angle"() -> (w364:dbl)
            "Gyro Angle 3" <- w364
            n251 = Wait Until Next ms Multiple(millisecond multiple=u32 20) -> ()  [unwired: 1 out]
            n252 = call <vilib>:"WPI_EncoderGet.vi"("EncoderDevRef"=w356) -> ("Distance"=w358:dbl)  [unwired: 5 in, 5 out]
            n253 = call <vilib>:"WPI_CANTalonSRX_GetStatus.vi"("CAN Talon SRX Ref"=w355) -> ("Talon SRX Status"=w366:T11)  [unwired: 8 in, 2 out]
            n254 = Subtract(x=w358, y=w357) -> (x-y=w354:dbl)
            "Distance 1" <- w354
            n255 = Unbundle By Name(w366) -> ("Current"=→"drive current 2":dbl)
            n256 = Absolute Value(x=w354) -> (abs(x)=w352:dbl)
            n257 = Greater?(x=w352, y=50.0) -> (0:w351:bool)
            n258 = case shown="True" w351 {
              frame False {
              }
              frame True {
                n259 = global write "Robot Global Data.vi" "x"(0.3 ("x")) -> ()
              }
            }
            n260 = call "Elapsed Time2"() -> ("Time has Elapsed"=w360:bool)  [unwired: 12 in, 7 out]
            n261 = call-poly <vilib>:"PID.vi"("output range"=cluster{"output high":dbl, "output low":dbl} {"output high"=0.6, "output low"=-0.6}, "PID gains"=T2 {"proportional gain (Kc)"=0.018, "integral time (Ti, min)"=0.0, "derivative time (Td, min)"=0.0}, "process variable"=w364, "setpoint"=w368) -> ("output"=w362:dbl)  [unwired: 6 in, 1 out]
            n262 = Greater Or Equal?(x=w352, y=80.0) -> (x >= y?=w361:bool)
            n263 = Or(x=w360, y=w361) -> (x .or. y?=w359:bool)
            n264 = global write "Robot Global Data.vi" "z"(w362) -> ()
          }
        }
        frame #3 {
          n265 = Add(x=0.0, y=w382) -> (x+y=w383:dbl)
          n266 = call <vilib>:"WPI_EncoderRefNum Registry Get.vi"("refnum name"="BL Encoder") -> ("EncoderDevRef"=w377:T3)  [unwired: 9 in, 1 out]
          n267 = global write "Robot Global Data.vi" "y"(0.5 ("y")) -> ()
          n268 = global write "Robot Global Data.vi" "x"(0.0 ("x")) -> ()
          n269 = global write "Robot Global Data.vi" "z"(0.0 ("z")) -> ()
          n270 = call <vilib>:"WPI_EncoderGet.vi"("EncoderDevRef"=w377) -> ("Distance"=w372:dbl, "EncoderDevRef"=w375:T3)  [unwired: 5 in, 4 out]
          n271 = call <vilib>:"WPI_MotorControlRefNum Registry Get.vi"("refnum name"="FR Drive Motor") -> ("MotorControlDevRef"=w374:T7)  [unwired: 9 in, 1 out]
          n272 = Wait (ms)(milliseconds to wait=u32 10) -> ()  [unwired: 1 out]
        }
        frame #4 {
          n273 = while {
            tunnel: w387 -> [w412]
            tunnel: w389 -> [w409]
            tunnel: w386 -> [w405]
            tunnel: w385 -> [w392]
            stop <- w401 stop-if-true
            n274 = call <vilib>:"WPI_CANTalonSRX_GetStatus.vi"("CAN Talon SRX Ref"=w405) -> ("Talon SRX Status"=w406:T11)  [unwired: 8 in, 2 out]
            n275 = call <vilib>:"WPI_EncoderGet.vi"("EncoderDevRef"=w412) -> ("Distance"=w393:dbl)  [unwired: 5 in, 5 out]
            n276 = Wait Until Next ms Multiple(millisecond multiple=u32 20) -> ()  [unwired: 1 out]
            n277 = global read "Robot Global Data.vi" "Gyro Angle"() -> (w395:dbl)
            "Gyro Angle 4" <- w395
            n278 = Subtract(x=w393, y=w392) -> (x-y=w394:dbl)
            "Distance 2" <- w394
            n279 = call "Elapsed Time8"() -> ("Elapsed Time (s)"=→"Elapsed Time (s) 2":dbl, "Time has Elapsed"=w400:bool)  [unwired: 12 in, 6 out]
            n280 = Unbundle By Name(w406) -> ("Current"=w390:dbl)
            "Current 2" <- w390
            n281 = Absolute Value(x=w394) -> (abs(x)=w408:dbl)
            n282 = call-poly <vilib>:"PID.vi"("output range"=cluster{"output high":dbl, "output low":dbl} {"output high"=0.6, "output low"=-0.6}, "PID gains"=T2 {"proportional gain (Kc)"=0.018, "integral time (Ti, min)"=0.0, "derivative time (Td, min)"=0.0}, "process variable"=w395, "setpoint"=w409) -> ("output"=w396:dbl)  [unwired: 6 in, 1 out]
            n283 = Greater Or Equal?(x=w390, y=20.0) -> (x >= y?=w402:bool)
            n284 = Greater Or Equal?(x=w408, y=50.0) -> (x >= y?=w403:bool)
            n285 = Compound Arithmetic op=OR(w400, w402, w403) -> (w401:bool)
            n286 = global write "Robot Global Data.vi" "z"(w396) -> ()
            n287 = call-poly <vilib>:"NT Write Value.vi"("Numeric"=w390, "Name"="BR Current") -> ()  [unwired: 9 in, 1 out]
            "Boolean 9" <- TRUE
            "Numeric 2" <- w409
          }
        }
        frame #5 {
          n288 = global write "Robot Global Data.vi" "Shoot"(TRUE ("Shoot")) -> ()
          n289 = Add(x=11.0, y=w417) -> (x+y=w416:dbl)
          n290 = global write "Robot Global Data.vi" "y"(0.0 ("y")) -> ()
          n291 = global write "Robot Global Data.vi" "x"(0.0 ("x")) -> ()
          n292 = global write "Robot Global Data.vi" "z"(0.0 ("z")) -> ()
          n293 = Wait (ms)(milliseconds to wait=u32 1500) -> ()  [unwired: 1 out]
        }
        frame #6 {
          n294 = while {
            tunnel: w421 -> [w431]
            stop <- w423 stop-if-true
            n295 = global read "Robot Global Data.vi" "Gyro Angle"() -> (w427:dbl)
            n296 = Wait Until Next ms Multiple(millisecond multiple=u32 20) -> ()  [unwired: 1 out]
            n297 = global write "Robot Global Data.vi" "Rot Pt Y"(18.0 ("x")) -> ()
            n298 = global write "Robot Global Data.vi" "Rot Pt X"(15.0 ("x")) -> ()
            n299 = Greater Or Equal?(x=w427, y=w431) -> (x >= y?=w424:bool)
            n300 = call "Elapsed Time9"() -> ("Time has Elapsed"=w422:bool)  [unwired: 12 in, 7 out]
            n301 = Or(x=w422, y=w424) -> (x .or. y?=w423:bool)
            n302 = call-poly <vilib>:"PID.vi"("output range"=cluster{"output high":dbl, "output low":dbl} {"output high"=0.4, "output low"=-0.4}, "PID gains"=T2 {"proportional gain (Kc)"=0.015, "integral time (Ti, min)"=0.035, "derivative time (Td, min)"=0.0} ("PID gains 2"), "process variable"=w427, "setpoint"=w431) -> ("output"=w425:dbl)  [unwired: 6 in, 1 out]
            n303 = global write "Robot Global Data.vi" "z"(w425) -> ()
            "Boolean 2" <- TRUE
          }
        }
        frame #7 {
          n304 = global write "Robot Global Data.vi" "Feed Shooter"(TRUE ("Feed Shooter")) -> ()
          n305 = global write "Robot Global Data.vi" "Shoot"(TRUE ("Shoot")) -> ()
          n306 = global write "Robot Global Data.vi" "z"(0.0 ("z")) -> ()
          n307 = Wait (ms)(milliseconds to wait=u32 12000) -> ()  [unwired: 1 out]
        }
        frame #8 {
          n308 = global write "Robot Global Data.vi" "Feed Shooter"(FALSE ("Feed Shooter")) -> ()
          n309 = global write "Robot Global Data.vi" "Shoot"(FALSE ("Shoot")) -> ()
          n310 = global write "Robot Global Data.vi" "y"(0.0 ("y")) -> ()
          n311 = global write "Robot Global Data.vi" "x"(0.0 ("x")) -> ()
          n312 = global write "Robot Global Data.vi" "z"(0.0 ("z")) -> ()
        }
      }
    }
  }
